vi "Using IO Variable.vi"() -> ()   [LabVIEW 2020]
panel:
  out "error out 4":errorcluster
  out "DIO0":bool
  in  "DIO4":bool
  out "AO0":dbl
  out "error out 3":errorcluster
  out "Green ways":dbl
  in  "milliseconds to wait":u32
  in  "stop":bool
  out "error out 2":errorcluster
  out "AI1":dbl
  out "error out":errorcluster
  out "AI0":dbl
  in  "Common":dbl
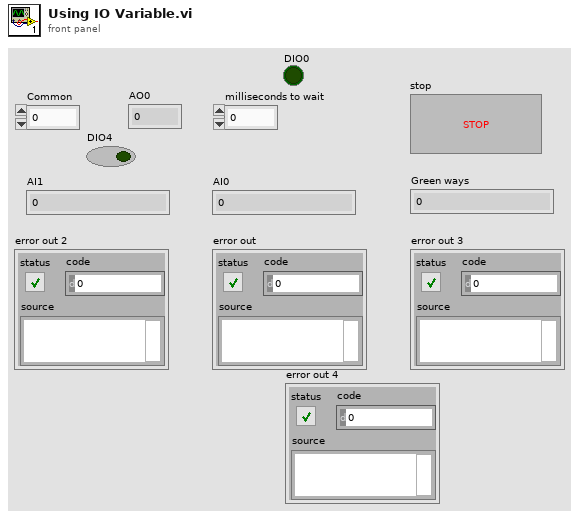
[diagram p1: front panel]
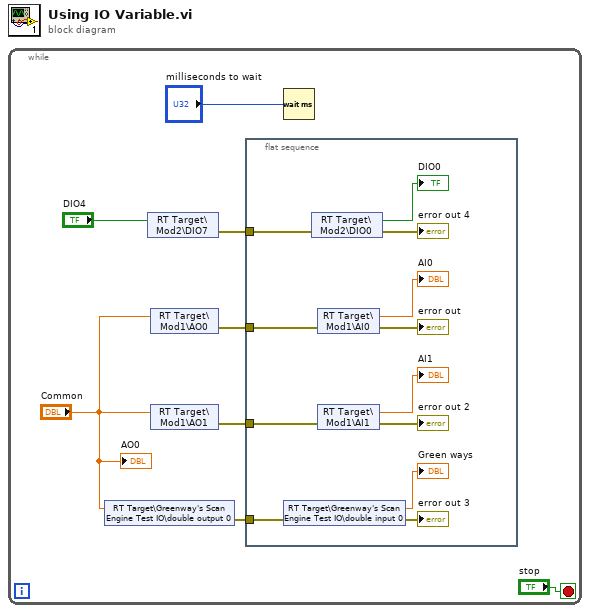
[diagram p0: block diagram]
diagram:
  n1 = while {
    stop <- "stop" stop-if-true
    n2 = shared-variable "RT Target\\Greenway's Scan Engine Test IO\\double output 0"("Common") -> (error out=w5:errorcluster)  [unwired: 1 in]
    n3 = shared-variable "RT Target\\Mod2\\DIO7"("DIO4") -> (error out=w1:errorcluster)  [unwired: 1 in]
    n4 = shared-variable "RT Target\\Mod1\\AO0"("Common") -> (error out=w3:errorcluster)  [unwired: 1 in]
    n5 = shared-variable "RT Target\\Mod1\\AO1"("Common") -> (error out=w7:errorcluster)  [unwired: 1 in]
    n6 = flat-sequence {
      tunnel: w7 -> [w18]
      tunnel: w5 -> [w17]
      tunnel: w3 -> [w14]
      tunnel: w1 -> [w11]
      frame #0 {
        n7 = shared-variable "RT Target\\Greenway's Scan Engine Test IO\\double input 0"(error in=w17) -> (→"Green ways":dbl, error out=→"error out 3":errorcluster)
        n8 = shared-variable "RT Target\\Mod2\\DIO0"(error in=w11) -> (→"DIO0":bool, error out=→"error out 4":errorcluster)
        n9 = shared-variable "RT Target\\Mod1\\AI0"(error in=w14) -> (→"AI0":dbl, error out=→"error out":errorcluster)
        n10 = shared-variable "RT Target\\Mod1\\AI1"(error in=w18) -> (→"AI1":dbl, error out=→"error out 2":errorcluster)
      }
    }
    n11 = Wait (ms)(milliseconds to wait="milliseconds to wait") -> ()  [unwired: 1 out]
    "AO0" <- "Common"
  }
